vi "Generate write queue item.vi"(8 "error in (no error)":errorcluster, 10 "Request ID":u64, 11 "CallRequest (MsgPack)":refnum<class "CallRequest (MsgPack).lvclass">) -> (0 "error out":errorcluster, 3 "Write queue item":T1)   [LabVIEW 2020, in "wamplv.lvlib" / "CallRequest (MsgPack).lvclass"]
uses:
  CallRequest (MsgPack).lvclass
  CallRequest (MsgPack).lvclass/CallRequest (MsgPack).ctl
  MessagePack/MsgPackString/MsgPackString.lvclass
  MessagePack/MessagePack.lvlib
  MessagePack/MsgPackArray/MsgPackArray.lvclass
  fd5207c4-3310-47b0-9035-a65521896721.vi
  TypeDefs/WAMP Message Codes.ctl
  wamplv.lvlib
  76aed925-7ccf-4c0a-adcf-a08a1e6fedd8.vi
  e0a91668-5700-44b2-bcc5-b581279df845.vi
  C:/local/wamplv/MessagePack/IMsgPackContainer/IMsgPackContainer.lvclass
  C:/local/wamplv/MessagePack/IMessagePackObject/IMessagePackObject.lvclass
  C:/local/wamplv/MessagePack/MsgPackArray/MsgPackArray.lvclass
  MessagePack/MsgPackMap/MsgPackMap.lvclass
  C:/local/wamplv/MessagePack/MsgPackMap/MsgPackMap.lvclass
  MessagePack/MessagePackNumeric/MessagePackNumeric.lvclass
  C:/local/wamplv/MessagePack/MessagePackNumeric/MessagePackNumeric.lvclass
  C:/local/wamplv/MessagePack/MsgPackString/MsgPackString.lvclass
  TypeDefs/Transport type.ctl
  WAMP Client/Private/TypeDef/Write queue item.ctl
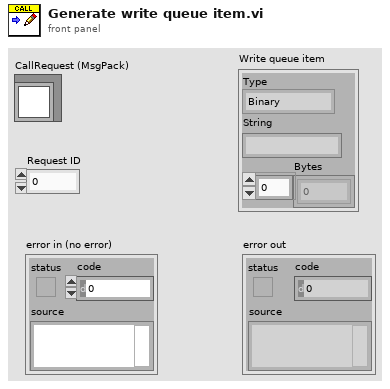
[diagram p1: front panel]
types:
  T1 = typedef "wamplv.lvlib/Write queue item.ctl" = cluster{"Type":T2, "String":string, "Bytes":u8[]}
  T2 = typedef "wamplv.lvlib/Transport type.ctl" = enum16{"Binary", "Text"}
  T3 = typedef "wamplv.lvlib/WAMP Message Codes.ctl" = u16
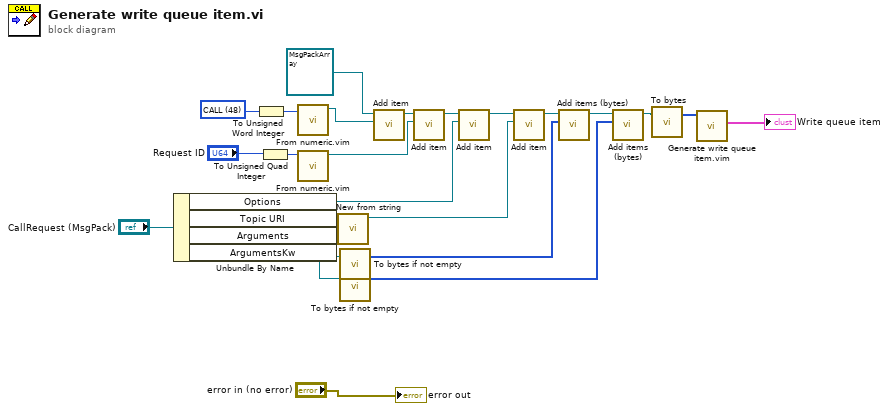
[diagram p0: block diagram]
diagram:
  w16 = T3 48 items=["HELLO"=1, "WELCOME"=2, "ABORT"=3, "GOODBYE"=6, "ERROR"=8, "PUBLISH"=16, "PUBLISHED"=17, "SUBSCRIBE"=32, "SUBSCRIBED"=33, "UNSUBSCRIBE"=34, "UNSUBSCRIBED"=35, "EVENT"=36, "CALL"=48, "RESULT"=59, "REGISTER"=64, "REGISTERED"=65, "UNREGISTER"=66, "UNREGISTERED"=67, "INVOCATION"=68, "YIELD"=70] ("Message Codes")
  n1 = Unbundle By Name("CallRequest (MsgPack)") -> ("Options"=w6:refnum<class "MsgPackMap.lvclass">, "Topic URI"=w24:string, "Arguments"=w23:refnum<class "MsgPackArray.lvclass">, "ArgumentsKw"=w22:refnum<class "MsgPackMap.lvclass">)
  n2 = To Unsigned Word Integer(number=w16) -> (unsigned 16bit integer=w15:T3)
  n3 = To Unsigned Quad Integer(1:"Request ID") -> (0:w17:u64)
  n4 = call "From numeric.vim"("Number"=w15) -> ("MessagePackNumeric out"=w13:refnum<class "MessagePackNumeric.lvclass">)  [unwired: 10 in]
  n5 = call "From numeric.vim"("Number"=w17) -> ("MessagePackNumeric out"=w11:refnum<class "MessagePackNumeric.lvclass">)  [unwired: 10 in]
  n6 = call "New from string.vi"("String"=w24) -> ("output cluster"=w21:refnum<class "MsgPackString.lvclass">)  [unwired: 10 in]
  n7 = call "To bytes if not empty.vi"("MessagePack.lvlib:IMsgPackContainer.lvclass"=w23) -> ("Array"=w19:u8[])  [unwired: 2 in]
  n8 = call "To bytes if not empty.vi"("MessagePack.lvlib:IMsgPackContainer.lvclass"=w22) -> ("Array"=w10:u8[])  [unwired: 2 in]
  n9 = call "Add item.vi"("wamplv.lvlib:IMessagePackObject.lvclass"=w13, "MsgPackArray in"=refnum<class "MsgPackArray.lvclass"> refnum ("MessagePack.lvlib:MsgPackArray.lvclass")) -> ("MsgPackArray out"=w12:refnum<class "MsgPackArray.lvclass">)  [unwired: 9 in]
  n10 = call "Add item.vi"("wamplv.lvlib:IMessagePackObject.lvclass"=w11, "MsgPackArray in"=w12) -> ("MsgPackArray out"=w8:refnum<class "MsgPackArray.lvclass">)  [unwired: 9 in]
  n11 = call "Add item.vi"("wamplv.lvlib:IMessagePackObject.lvclass"=w6, "MsgPackArray in"=w8) -> ("MsgPackArray out"=w7:refnum<class "MsgPackArray.lvclass">)  [unwired: 9 in]
  n12 = call "Add item.vi"("wamplv.lvlib:IMessagePackObject.lvclass"=w21, "MsgPackArray in"=w7) -> ("MsgPackArray out"=w20:refnum<class "MsgPackArray.lvclass">)  [unwired: 9 in]
  n13 = call "Add items (bytes).vi"("Array"=w19, "MsgPackArray in"=w20) -> ("MsgPackArray out"=w18:refnum<class "MsgPackArray.lvclass">)  [unwired: 9 in]
  n14 = call "Add items (bytes).vi"("Array"=w10, "MsgPackArray in"=w18) -> ("MsgPackArray out"=w9:refnum<class "MsgPackArray.lvclass">)  [unwired: 9 in]
  n15 = call-dynamic "To bytes.vi"("MsgPackArray in"=w9) -> ("Array"=w3:u8[])  [unwired: 2 in]
  n16 = call "Generate write queue item.vim"("Input"=w3) -> ("Ouput"=→"Write queue item":T1)  [unwired: 2 in]
  "error out" <- "error in (no error)"
